vi "Script Find current Constants.vi"(8 "error in":errorcluster, 11 "Library in":refnum<vi>) -> (0 "error out":errorcluster, 2 "Constant VIs":string[](array[string]), 3 "Library out":refnum<vi>)   [LabVIEW 2019, in "Panther Dashboard.lvlib"]
uses:
  Panther Dashboard.lvlib
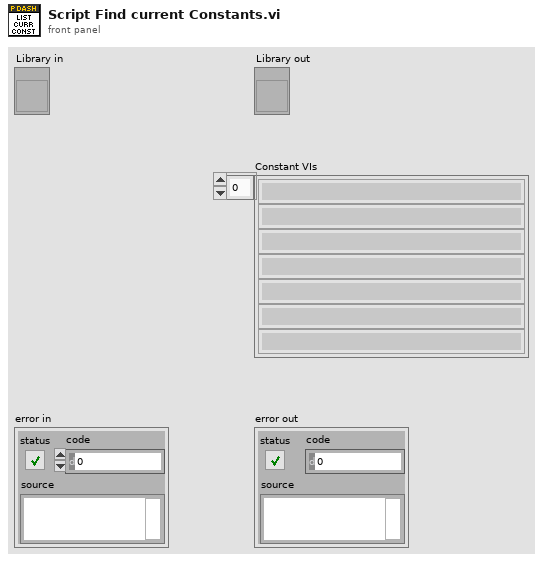
[diagram p1: front panel]
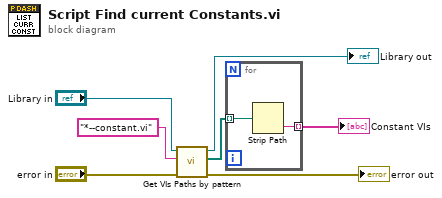
[diagram p0: block diagram]
diagram:
  n1 = call "Get VIs Paths by pattern.vi"("error in (no error)"="error in", "pattern"="*--constant.vi", "Library in"="Library in") -> ("error out"=→"error out":errorcluster, "All Files in Dir"=w1:path[], "Library out"=→"Library out":refnum<vi>)  [unwired: 6 in]
  n2 = for {
    tunnel: w1 -> [w9] mode=indexing
    tunnel: [w8] -> w5 mode=indexing
    n3 = Strip Path(path=w9) -> (name=w8:string)  [unwired: 1 out]
  }
  "Constant VIs" <- w5
